vi "Script VIs.vi"(6 "VI Refs":T3, 8 "error in":errorcluster, 9 "Msg Output Terminal Attributes":T1, 10 "Msg Terminal Attributes":T1) -> (0 "error out":errorcluster)   [LabVIEW 2025, in "_Msg Rescript.lvlib" / "_Msg Rescript.lvclass"]
uses:
  _Msg Rescript.lvclass
  VI Refs.ctl
  Terminal Attributes.ctl
  Attributes.ctl
  <vilib>/Utility/traverseref.llb/TRef TravTarget.ctl
  _Msg Rescript.lvclass/_Msg Rescript.ctl
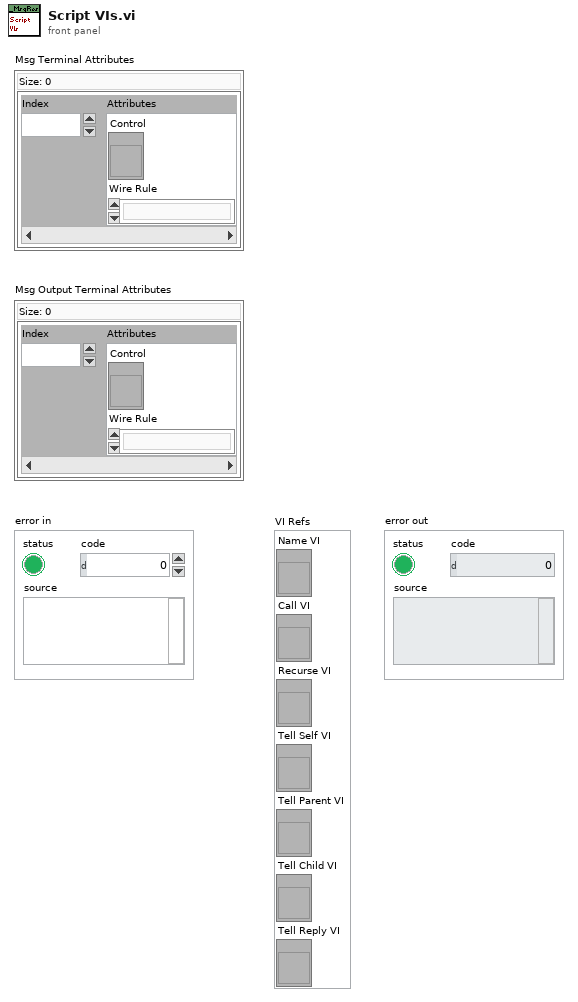
[diagram p1: front panel]
types:
  T1 = typedef "_Msg Rescript.lvlib/_Msg Rescript.lvclass/Terminal Attributes.ctl" = map{i32, T2}
  T2 = typedef "_Msg Rescript.lvlib/_Msg Rescript.lvclass/Attributes.ctl" = cluster{"Control":refnum<vi>, "Wire Rule":enum16{"Invalid Wire Rule", "Required", "Recommended", "Optional", "Dynamic Dispatch"}}
  T3 = typedef "_Msg Rescript.lvlib/_Msg Rescript.lvclass/VI Refs.ctl" = cluster{"Name VI":refnum<vi>, "Call VI":refnum<vi>, "Recurse VI":refnum<vi>, "Tell Self VI":refnum<vi>, "Tell Parent VI":refnum<vi>, "Tell Child VI":refnum<vi>, "Tell Reply VI":refnum<vi>}
  T4 = typedef "TRef TravTarget.ctl" = enum16{"FP", "BD", "Other"}
  T5 = enum16{"Invalid Wire Rule", "Required", "Recommended", "Optional", "Dynamic Dispatch"}
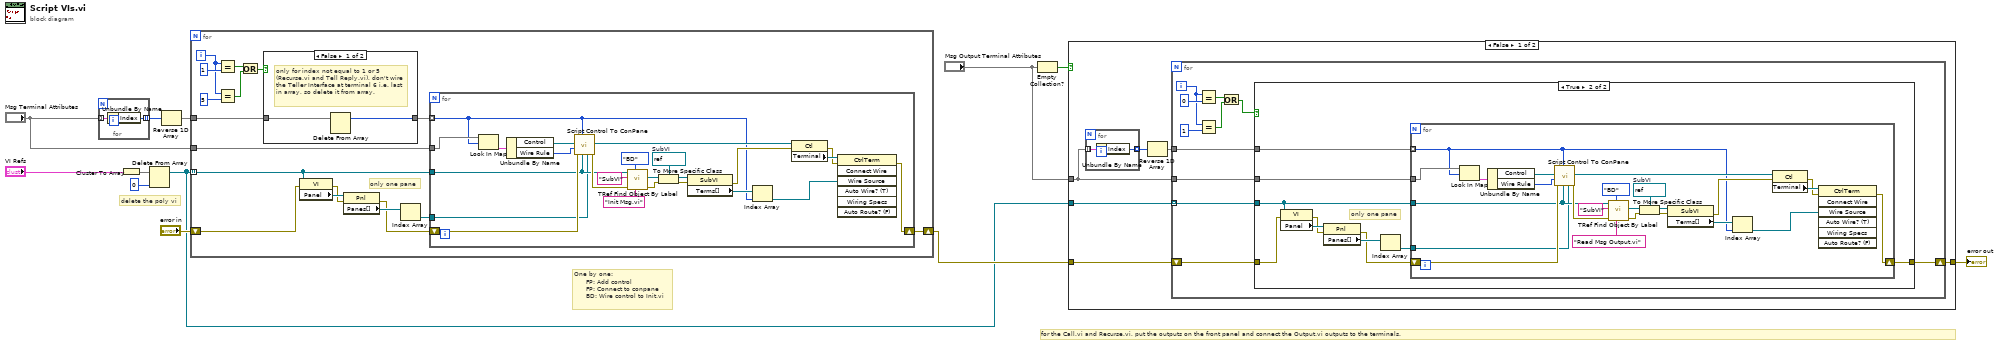
[diagram p0: block diagram]
diagram:
  # "delete the poly vi"
  # "for the Call.vi and Recurse.vi, put the outputs on the front panel and connect the Output.vi outputs to the terminals."
  # "One by one:\n      FP: Add control\n      FP: Connect to conpane\n      BD: Wire control to Init.vi"
  n1 = for {
    tunnel: "Msg Terminal Attributes" -> [w14] mode=indexing
    tunnel: [w13] -> w12 mode=indexing
    n2 = Unbundle By Name(w14) -> ("Index"=w13:i32)
  }
  n3 = Cluster To Array(cluster="VI Refs") -> (array=w4:refnum<vi>[])
  n4 = Delete From Array(array=w4, index=0) -> (array with subset deleted=w3:refnum<vi>[])  [unwired: 1 in, 1 out]
  n5 = Reverse 1D Array(array=w12) -> (reversed array=w11:i32[])
  n6 = for {
    tunnel: w11 -> [w21]
    tunnel: "Msg Terminal Attributes" -> [w31]
    shift-right: [w29] -> w7
    shift-left: "error in" -> [w30]
    tunnel: w3 -> [w27] mode=indexing
    i -> [w15]
    # "only one pane"
    n7 = Equal?(x=w15, y=1) -> (x = y?=w19:bool)
    n8 = Equal?(x=w15, y=5) -> (x = y?=w16:bool)
    n9 = Or(x=w19, y=w16) -> (x .or. y?=w18:bool)
    n10 = case shown="False" w18 {
      tunnel: w21 -> [w33 w34]
      tunnel: [w32 w34] -> w20
      frame False {
        # "only for index not equal to 1 or 5 (Recurse.vi and Tell Reply.vi), don't wire the Teller Interface at terminal 6 i.e. last in array, so delete it from array."
        n11 = Delete From Array(array=w33) -> (array with subset deleted=w32:i32[])  [unwired: 2 in, 1 out]
      }
      frame True {
      }
    }
    n12 = property class="VI"(reference=w27, error in=w30) -> (error out=w24:errorcluster, "Panel"=w26:refnum<vi>)  [unwired: 1 out]
    n13 = property class="Pnl"(reference=w26, error in=w24) -> (error out=w23:errorcluster, "Panes[]"=w25:refnum<vi>[])  [unwired: 1 out]
    n14 = Index Array(array=w25) -> (element=w22:refnum<vi>)  [unwired: 1 in]
    n15 = for {
      tunnel: w20 -> [w35] mode=indexing
      tunnel: w31 -> [w38]
      tunnel: w22 -> [w40]
      tunnel: w27 -> [w41]
      shift-right: [w56] -> w29
      shift-left: w23 -> [w44]
      w54 = refnum<vi> refnum  # SubVI
      n16 = Look In Map(map=w38, key=w35) -> (value=w39:T2)  [unwired: 1 in, 1 out]
      n17 = Unbundle By Name(w39) -> ("Control"=w37:refnum<vi>, "Wire Rule"=w36:T5)
      n18 = call "Script Control To ConPane.vi"("Pane"=w40, "VI Ref"=w41, "Terminal Index"=w35, "error in"=w44, "Wire Rule"=w36, "Control"=w37) -> ("error out"=w43:errorcluster, "Control"=w42:refnum<vi>)  [unwired: 4 in]
      n19 = call <vilib>:"TRef Find Object By Label.vi"("Label"="Init Msg.vi", "Traverse Target"=TRef_TravTarget."BD", "error in (no error)"=w43, "Class Name"="SubVI", "VI Ref"=w41) -> ("error out"=w53:errorcluster, "Found Obj Ref"=w48:refnum<vi>)  [unwired: 3 in, 2 out]
      n20 = To More Specific Class(target class=w54, reference=w48, error in=w53) -> (specific class reference=w51:refnum<vi>, error out=w50:errorcluster)
      n21 = property class="SubVI"(reference=w51, error in=w50) -> (error out=w45:errorcluster, "Terms[]"=w49:refnum<vi>[])  [unwired: 1 out]
      n22 = Index Array(array=w49, index=w35) -> (element=w46:refnum<vi>)
      n23 = property class="Ctl"(reference=w42, error in=w45) -> (error out=w57:errorcluster, "Terminal"=w58:refnum<vi>)  [unwired: 1 out]
      n24 = invoke class="CtrlTerm" method="Connect Wire"(reference=w58, error in=w57, "Wire Source"=w46) -> (error out=w56:errorcluster)  [unwired: 4 in, 6 out]
    }
  }
  n25 = Empty Collection?(1:"Msg Output Terminal Attributes") -> (0:w8:bool)
  n26 = case shown="False" w8 {
    tunnel: w3 -> [w64 _]
    tunnel: "Msg Output Terminal Attributes" -> [w62 _]
    tunnel: w7 -> [w60 w113]
    tunnel: [w59 w113] -> w6
    frame False {
      n27 = for {
        tunnel: w62 -> [w66] mode=indexing
        tunnel: [w65] -> w63 mode=indexing
        n28 = Unbundle By Name(w66) -> ("Index"=w65:i32)
      }
      n29 = Reverse 1D Array(array=w63) -> (reversed array=w61:i32[])
      n30 = for {
        tunnel: w61 -> [w68]
        tunnel: w62 -> [w77]
        shift-right: [w75] -> w59
        shift-left: w60 -> [w76]
        tunnel: w64 -> [w73] mode=indexing
        i -> [w69]
        n31 = Equal?(x=w69, y=0) -> (x = y?=w72:bool)
        n32 = Equal?(x=w69, y=1) -> (x = y?=w70:bool)
        n33 = Or(x=w72, y=w70) -> (x .or. y?=w67:bool)
        n34 = case shown="True" w67 {
          tunnel: w77 -> [_ w88]
          tunnel: w76 -> [w78 w87]
          tunnel: [w78 w86] -> w75
          tunnel: w73 -> [_ w85]
          tunnel: w68 -> [_ w79]
          frame False {
          }
          frame True {
            # "only one pane"
            n35 = property class="VI"(reference=w85, error in=w87) -> (error out=w82:errorcluster, "Panel"=w84:refnum<vi>)  [unwired: 1 out]
            n36 = property class="Pnl"(reference=w84, error in=w82) -> (error out=w81:errorcluster, "Panes[]"=w83:refnum<vi>[])  [unwired: 1 out]
            n37 = Index Array(array=w83) -> (element=w80:refnum<vi>)  [unwired: 1 in]
            n38 = for {
              tunnel: w79 -> [w89] mode=indexing
              tunnel: w88 -> [w92]
              tunnel: w80 -> [w94]
              tunnel: w85 -> [w95]
              shift-right: [w110] -> w86
              shift-left: w81 -> [w98]
              w108 = refnum<vi> refnum  # SubVI
              n39 = Look In Map(map=w92, key=w89) -> (value=w93:T2)  [unwired: 1 in, 1 out]
              n40 = Unbundle By Name(w93) -> ("Control"=w91:refnum<vi>, "Wire Rule"=w90:T5)
              n41 = call "Script Control To ConPane.vi"("Pane"=w94, "VI Ref"=w95, "Terminal Index"=w89, "error in"=w98, "Wire Rule"=w90, "Control"=w91) -> ("error out"=w97:errorcluster, "Control"=w96:refnum<vi>)  [unwired: 4 in]
              n42 = call <vilib>:"TRef Find Object By Label.vi"("Label"="Read Msg Output.vi", "Traverse Target"=TRef_TravTarget."BD", "error in (no error)"=w97, "Class Name"="SubVI", "VI Ref"=w95) -> ("error out"=w107:errorcluster, "Found Obj Ref"=w102:refnum<vi>)  [unwired: 3 in, 2 out]
              n43 = To More Specific Class(target class=w108, reference=w102, error in=w107) -> (specific class reference=w105:refnum<vi>, error out=w104:errorcluster)
              n44 = property class="SubVI"(reference=w105, error in=w104) -> (error out=w99:errorcluster, "Terms[]"=w103:refnum<vi>[])  [unwired: 1 out]
              n45 = Index Array(array=w103, index=w89) -> (element=w100:refnum<vi>)
              n46 = property class="Ctl"(reference=w96, error in=w99) -> (error out=w111:errorcluster, "Terminal"=w112:refnum<vi>)  [unwired: 1 out]
              n47 = invoke class="CtrlTerm" method="Connect Wire"(reference=w112, error in=w111, "Wire Source"=w100) -> (error out=w110:errorcluster)  [unwired: 4 in, 6 out]
            }
          }
        }
      }
    }
    frame True {
    }
  }
  "error out" <- w6
